vi "3.2.0 Kalman Control Input Matrix B.vi"(1 "State Vector X":T1) -> (0 "Real Matrix":T2)   [LabVIEW 2010]
uses:
  <vilib>/Analysis/Matrix/Datatypes/RealMatrix.ctl
  4-High Neurons/4.2/4.2.0 Kalman State.ctl
  <vilib>/Analysis/Matrix/Numeric/Conversions/Array To Matrix - RA2.vi
  <vilib>/Analysis/Matrix/NI_Matrix.lvlib
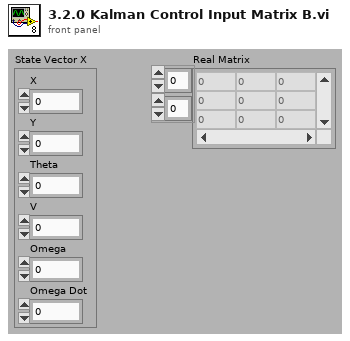
[diagram p1: front panel]
types:
  T1 = typedef "4.2.0 Kalman State.ctl" = cluster{"X":dbl, "Y":dbl, "Theta":dbl, "V":dbl, "Omega":dbl, "Omega Dot":dbl}
  T2 = typedef "NI_Matrix.lvlib/RealMatrix.ctl" = dbl[][]
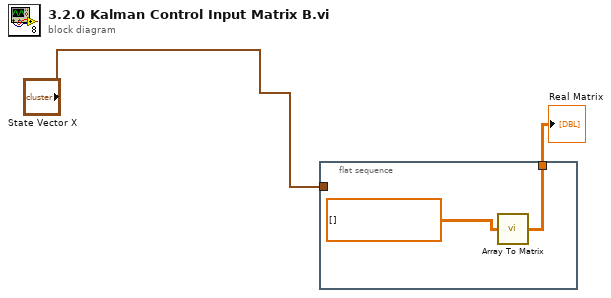
[diagram p0: block diagram]
diagram:
  n1 = flat-sequence {
    tunnel: "State Vector X" -> [_]
    tunnel: [w3] -> w2
    frame #0 {
      n2 = call-poly <vilib>:"Array To Matrix.vi"("Real 2D Array"=dbl[][] []) -> ("Real Matrix"=w3:T2)
    }
  }
  "Real Matrix" <- w2
